vi "auto save.vi"() -> ()   [LabVIEW 2020]
uses:
  b99c64d7-138e-4fcd-9fd2-310e4f16eab7.vi
  <vilib>/Comparison/Equal/Equal Functor/Equal Functor.lvclass
panel:
  out "Array 2":i32[](array[numeric])
  out "Array":i32[](array[numeric])
  out "output array":i32[](array[numeric])
  out "x+y":dbl[][](array[numeric])
  out "Numeric 6":i32
  out "Last val 10":i32
  out "Last val 9":i32[](array[numeric])
  out "Numeric 5":i32
  out "Last val 8":i32
  out "Last val 7":i32[](array[numeric])
  out "Numeric 4":i32
  out "Last val 6":i32
  out "Last val 5":i32[](array[numeric])
  out "Numeric 3":i32
  out "Last val 4":i32
  out "Last val 3":i32[](array[numeric])
  out "Last val 2":i32[](array[numeric])
  out "Last val":i32
  out "Sum":i32
  out "Numeric 2":i32
  out "min index(es)":i32
  out "min value":i32
  out "max index(es)":i32
  out "max value":i32
  in  "stop":bool
  out "Numeric":i32
  out "deleted portion":i32
  out "array w/ subset deleted":i32[](array[numeric])
  out "index of element":i32
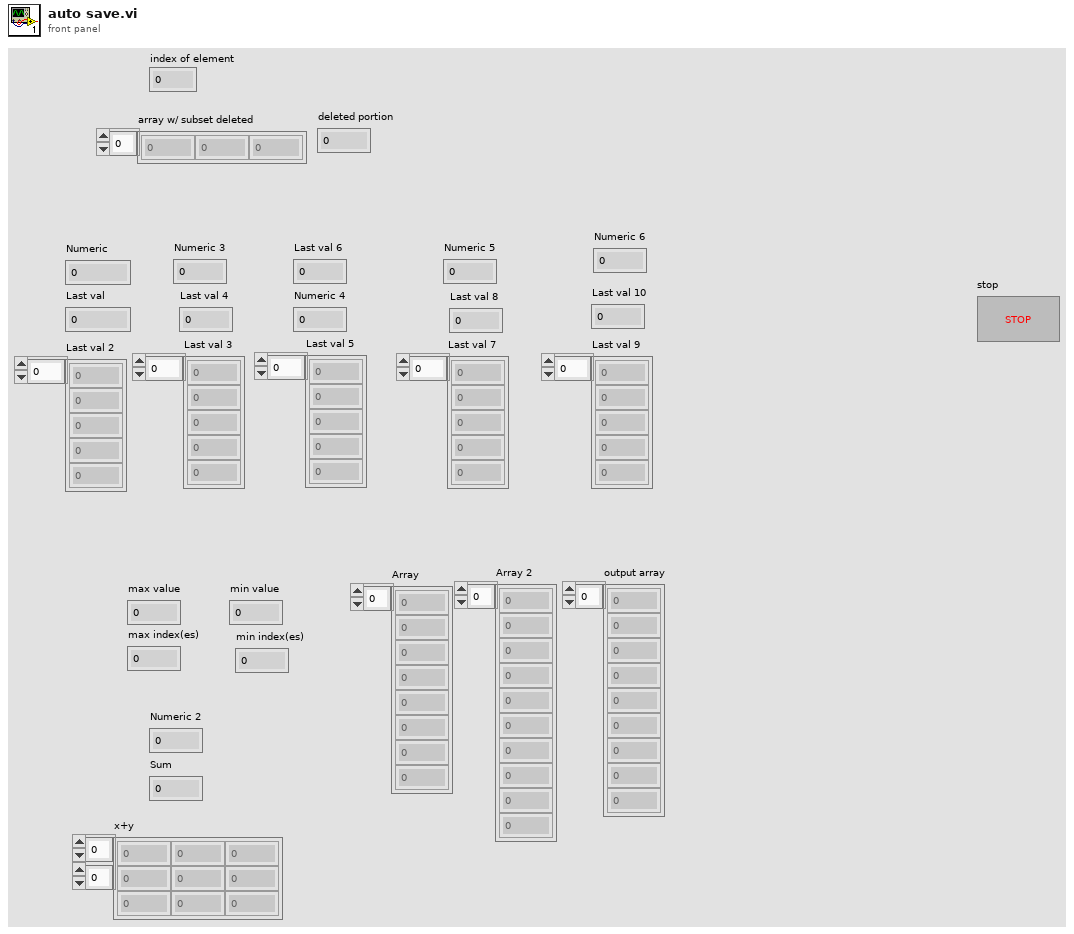
[diagram p1: front panel]
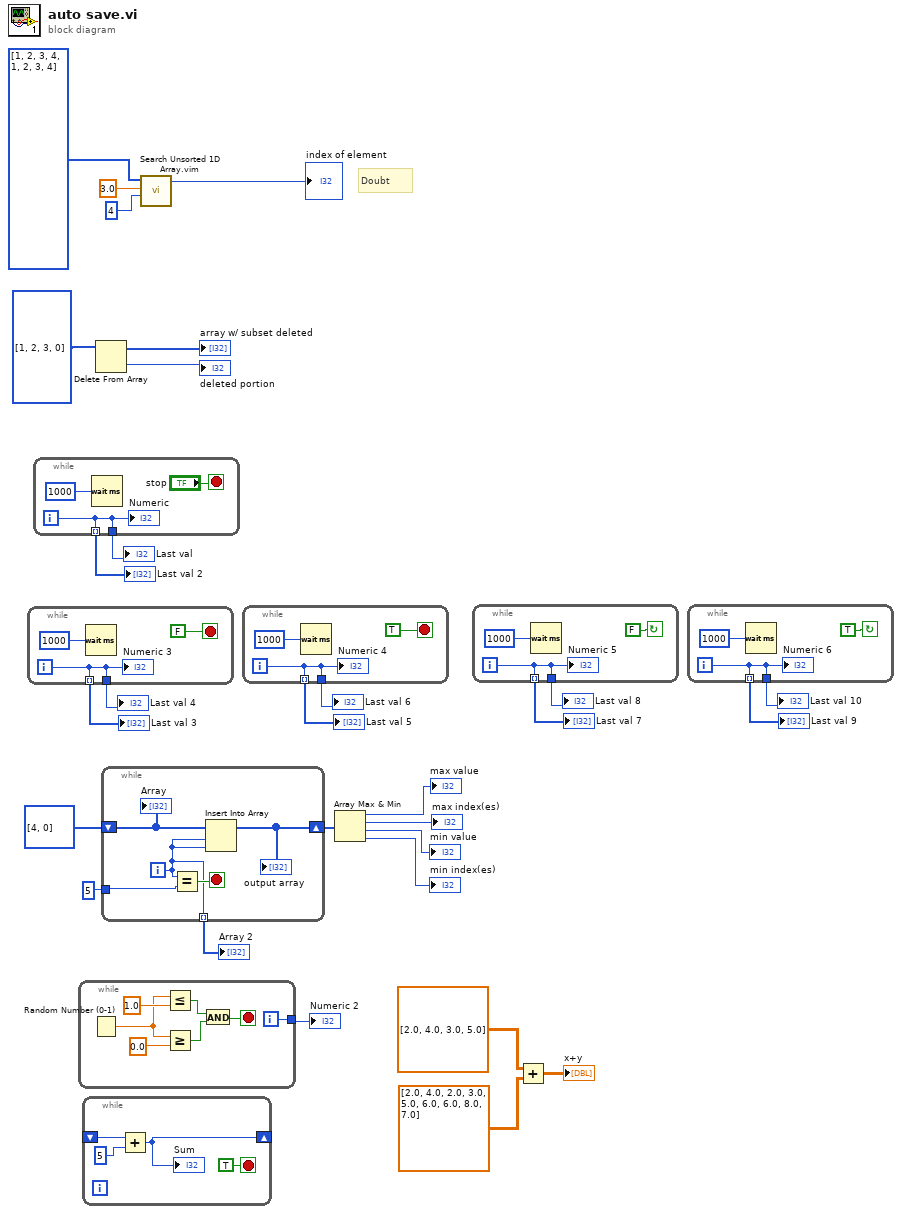
[diagram p0: block diagram]
diagram:
  # "Doubt"
  n1 = while {
    tunnel: [w31] -> w12
    tunnel: [w31] -> w13 mode=indexing
    i -> [w31]
    stop <- FALSE stop-if-true
    n2 = Wait (ms)(milliseconds to wait=u32 1000 ("millisecond timer value")) -> ()  [unwired: 1 out]
    "Numeric 3" <- w31
  }
  "Last val 4" <- w12
  "Last val 3" <- w13
  n3 = while {
    tunnel: [w33] -> w15
    tunnel: [w33] -> w14 mode=indexing
    i -> [w33]
    stop <- "stop" stop-if-true
    n4 = Wait (ms)(milliseconds to wait=u32 1000 ("millisecond timer value")) -> ()  [unwired: 1 out]
    "Numeric" <- w33
  }
  "Last val" <- w15
  "Last val 2" <- w14
  n5 = while {
    tunnel: [w36] -> w5
    i -> [w36]
    stop <- w37 stop-if-true
    n6 = Random Number (0-1)() -> (number: 0 to 1=w38:dbl)
    n7 = Less Or Equal?(x=w38, y=1.0) -> (x <= y?=w40:bool)
    n8 = Greater Or Equal?(x=w38, y=0.0) -> (x >= y?=w39:bool)
    n9 = And(x=w40, y=w39) -> (x .and. y?=w37:bool)
  }
  "Numeric 2" <- w5
  n10 = while {
    shift-right: [w44] -> _
    shift-left: _ -> [w45]
    stop <- TRUE stop-if-true
    n11 = Add(x=w45, y=5) -> (x+y=w44:i32)
    "Sum" <- w44
  }
  n12 = Delete From Array "Delete From Array"(array=i32[] [1, 2, 3, 0]) -> (deleted portion=→"deleted portion":i32, array with subset deleted=→"array w/ subset deleted":i32[])  [unwired: 2 in]
  n13 = while {
    tunnel: 5 -> [w50]
    shift-right: [w49] -> w20
    shift-left: i32[] [4, 0] -> [w47]
    tunnel: [w48] -> w1 mode=indexing
    i -> [w48]
    stop <- w51 stop-if-true
    n14 = Equal?(x=w48, y=w50) -> (x = y?=w51:bool)
    n15 = Insert Into Array "Insert Into Array"(array=w47, index=w48, new element=w48) -> (w49:i32[])
    "output array" <- w49
    "Array" <- w47
  }
  "Array 2" <- w1
  n16 = call "Search Unsorted 1D Array.vim"("start index (0)"=4, "element"=3.0, "unsorted 1D array"=i32[] [1, 2, 3, 4, 1, 2, 3, 4]) -> ("index of element"=→"index of element":i32)  [unwired: 8 in]
  n17 = while {
    tunnel: [w53] -> w11
    tunnel: [w53] -> w10 mode=indexing
    i -> [w53]
    stop <- TRUE stop-if-true
    n18 = Wait (ms)(milliseconds to wait=u32 1000 ("millisecond timer value")) -> ()  [unwired: 1 out]
    "Numeric 4" <- w53
  }
  "Last val 6" <- w11
  "Last val 5" <- w10
  n19 = Array Max & Min(array=w20) -> (max value=→"max value":i32, max index (indices)=→"max index(es)":i32, min value=→"min value":i32, min index (indices)=→"min index(es)":i32)
  n20 = while {
    tunnel: [w56] -> w9
    tunnel: [w56] -> w8 mode=indexing
    i -> [w56]
    stop <- FALSE continue-if-true
    n21 = Wait (ms)(milliseconds to wait=u32 1000 ("millisecond timer value")) -> ()  [unwired: 1 out]
    "Numeric 5" <- w56
  }
  "Last val 8" <- w9
  "Last val 7" <- w8
  n22 = Add(x=dbl[][] [[2.0, 4.0], [3.0, 5.0]], y=dbl[][] [[2.0, 4.0, 2.0], [3.0, 5.0, 6.0], [6.0, 8.0, 7.0]]) -> (x+y=→"x+y":dbl[][])
  n23 = while {
    tunnel: [w59] -> w6
    tunnel: [w59] -> w7 mode=indexing
    i -> [w59]
    stop <- TRUE continue-if-true
    n24 = Wait (ms)(milliseconds to wait=u32 1000 ("millisecond timer value")) -> ()  [unwired: 1 out]
    "Numeric 6" <- w59
  }
  "Last val 10" <- w6
  "Last val 9" <- w7
